vi "niFPGA U32 To SGL Cast.vi"(4 "x":u32 format="%.0x") -> (1 "y":sgl)   [LabVIEW 2017]
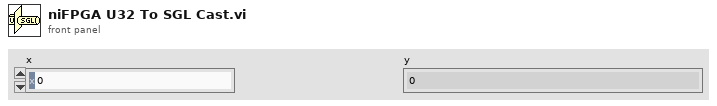
[diagram p1: front panel]
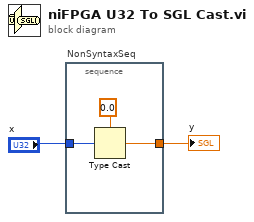
[diagram p0: block diagram]
diagram:
  n1 = stacked-sequence "NonSyntaxSeq" {
    tunnel: "x" -> [w4]
    tunnel: [w3] -> w1
    frame #0 {
      n2 = Type Cast(type=sgl 0.0, x=w4) -> (*(type *) &x=w3:sgl)
    }
  }
  "y" <- w1
